vi "Get All Elements.vi"(8 "error in":errorcluster, 10 "Section Node":refnum<k20>, 11 "Section Ref in":refnum<data-value>) -> (0 "error out":errorcluster, 3 "Section Ref out":refnum<data-value>)   [LabVIEW 2024, in "Config File Parser.lvlib" / "Section.lvclass"]
uses:
  Section.lvclass
  C:/dev/CD/CD 2.0/Config-File-Parser/Item/Item.lvclass
  <vilib>/xml/Close Reference(Node).vi
  <resource>/objmgr/DOMUserDefRef.rc
  Config File Parser.lvlib
  <vilib>/xml/NI_XML.lvlib
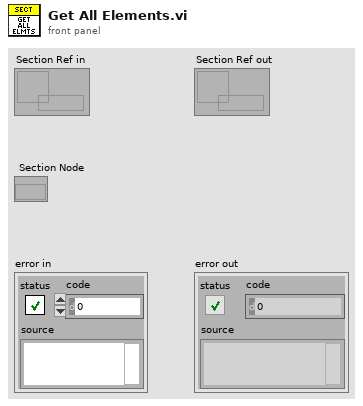
[diagram p1: front panel]
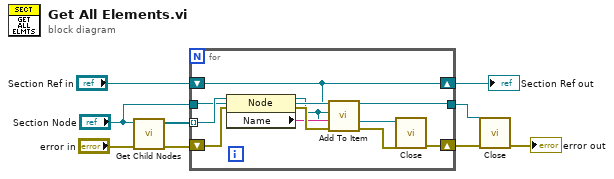
[diagram p0: block diagram]
diagram:
  n1 = call "Get Child Nodes.vi"("error in"="error in", "Node"="Section Node") -> ("error out"=w8:errorcluster, "Child Nodes"=w5:refnum<k20>[])  [unwired: 8 in]
  n2 = for {
    tunnel: w5 -> [w16] mode=indexing
    shift-right: [w11] -> w6
    shift-left: w8 -> [w18]
    tunnel: [w14] -> w3
    tunnel: "Section Node" -> [w14]
    shift-right: [w13] -> w1
    shift-left: "Section Ref in" -> [w13]
    n3 = property class="Node"(reference=w16, error in=w18) -> (reference out=w10:refnum<k20>, error out=w17:errorcluster, "Name"=w15:string)
    n4 = call "Add To Item.vi"("error in"=w17, "Item Name"=w15, "Item node"=w10, "Parent Item Ref in"=w13) -> ("error out"=w12:errorcluster)  [unwired: 6 in, 1 out]
    n5 = call-poly <vilib>:"Close.vi"("error in (no error)"=w12, "node"=w10) -> ("error out"=w11:errorcluster)  [unwired: 7 in]
  }
  "Section Ref out" <- w1
  n6 = call-poly <vilib>:"Close.vi"("error in (no error)"=w6, "node"=w3) -> ("error out"=→"error out":errorcluster)  [unwired: 7 in]
